vi "MultiChannelFeedback_test_no_before (Host).vi"(5 "RIO Device":T1="RIO0") -> ()   [LabVIEW 2016]
doc: "This VI will will initialize the FPGA VI and then continually read and convert single point values from 4 channels of an analog input module."
uses:
  <vilib>/userdefined/High Color/nirio_resource_hc.ctl
  <vilib>/rvi/Analysis/host/Butterworth/config/Butterworth Filter Order.ctl
  <vilib>/rvi/Analysis/host/Butterworth/config/Butterworth Filter Type.ctl
  <vilib>/FPGAPlugInAG/PXIe-7847R/niLvFpga_Open_PXIe-7847R.vi
  <vilib>/FPGAPlugInAG/PXIe-7847R/niLvFpga_Run_PXIe-7847R.vi
  <vilib>/rvi/Analysis/host/Butterworth/config/BwScaledCoefficients.vi
  <vilib>/Utility/error.llb/Error Cluster From Error Code.vi
  <vilib>/rvi/errors/niLvFpgaAdjustHostInterfaceError.vi
  <vilib>/Utility/file.llb/Read From Spreadsheet File (I64).vi
  <vilib>/FPGAPlugInAG/PXIe-7847R/niLvFpga_Close_PXIe-7847R.vi
  <vilib>/rvi/interface/nirviOpenFPGA/nirviOpenFPGA.xnode
  FPGA Bitfiles/Microspherefeedb_FPGATarget_MultiChannelfFee_-5RO42C0JZ0.lvbitx
  <vilib>/rvi/interface/nirviMethod/nirviMethod.xnode
  <vilib>/rvi/Analysis/host/Butterworth/XNode/ButterworthCoefficients.xnode
  <vilib>/rvi/interface/nirviReadWriteControl/nirviReadWriteControl.xnode
  <vilib>/rvi/interface/nirviCloseFPGA/nirviCloseFPGA.xnode
  NiFpgaLv.dll
  <vilib>/rvi/Analysis/host/Public/NI_FpgaMspHost.lvlib
panel:
  in  "ramp arb drive":bool
  in  "Write data to buffers":bool
  in  "z scale":fxp<+/-,33,17>=1.0
  in  "End value (ch1)":fxp<+/-,32,16>=1.0
  in  "Step (ch1)":fxp<+/-,32,16>=0.100006103515625
  in  "End value (ch0)":fxp<+/-,32,16>=1.0
  in  "Step (ch0)":fxp<+/-,32,16>=1.0
  in  "Delay Time (s)":dbl=0.001
  in  "gain (Z)":fxp<+/-,24,12>=1.0
  in  "steps per cycle":u16=40
  in  "gain (Y)":fxp<+/-,24,12>
  in  "gain (X)":fxp<+/-,24,12>=1.0
  in  "Buffer file path":path=path "C:/Users/UsphereLab/Documents/GitHub/Optlev/scriptssiny_buffer.txt"
  in  "Ramp":bool
  in  "End value power":i16=-800
  in  "Step power":i16=1
  in  "Delay Time (s) power":dbl=0.1 caption="Delay Time (s)"
  in  "LP FF Z":dbl=5000.0
  in  "LP FF Y":dbl=5000.0
  in  "LP FF X":dbl=5000.0
  in  "?":u16(ring)=2 items=["Both", "AOD", "Bead"]
  in  "?":u16(ring)=2 items=["Both", "AOD", "Bead"]
  out "Tot feedback + DC, Z":i16(graph)=80
  out "Individual feedback, Z":cluster{"fb_0":i16, "fb_d0":i16}(graph)={"fb_0"=99, "fb_d0"=99}
  out "AI 2":cluster{"AI1":i16, "AI4":i16}(graph)={"AI1"=301, "AI4"=301}
  out "EOM_amplitude_out":dbl=-6.999694842844065
  in  "EOM_offset (-10 to 10 V)":dbl
  in  "EOM_amplitude (-10 to 10 V)":dbl=-7.0
  in  "EOM_threshold (0 to 1), (2*thr - 1)*ampli":dbl=1.0
  in  "EOM reset":bool
  in  "Pg Y":fxp<+/-,24,12>
  in  "Ig Y":fxp<+/-,24,6>=3.814697265625e-06
  in  "Pg X":fxp<+/-,24,12>
  in  "Ig X":fxp<+/-,24,6>=-3.814697265625e-06
  in  "hp freq Y":dbl=1300.0
  in  "hp freq X":dbl=1300.0
  in  "lp freq X":dbl=1300.0
  in  "DC offset X":i16
  in  "Lower lim X":fxp<+/-,16,16>=-30000.0
  in  "Upper lim X":fxp<+/-,16,16>=30000.0
  in  "Dg X":fxp<+/-,24,12>=-3.5
  in  "X setpoint":i16
  in  "Update":bool
  in  "hp freq Z":dbl=3200.0
  in  "lp freq Y":dbl=1300.0
  in  "lp freq Z":dbl=3200.0
  in  "Count(usec)":u32=10
  in  "?":u16(ring)=2 items=["Both", "AOD", "Bead"]
  in  "?":u16(ring)=2 items=["Both", "AOD", "Bead"]
  in  "?":u16(ring)=2 items=["Both", "AOD", "Bead"]
  in  "?":u16(ring)=2 items=["Both", "AOD", "Bead"]
  in  "Ig Z":fxp<+/-,24,6>=3.814697265625e-06
  in  "DC offset Z":i16=-19
  in  "Lower lim Z":fxp<+/-,16,16>=-700.0
  in  "Upper lim Z":fxp<+/-,16,16>=1500.0
  in  "Dg Z":fxp<+/-,24,12>=3.0
  in  "Pg Z":fxp<+/-,24,12>=0.150146484375
  in  "Z setpoint":i16=300
  in  "Update":bool
  in  "Update":bool
  in  "DC offset Y":i16
  in  "Lower lim Y":fxp<+/-,16,16>=-30000.0
  in  "Upper lim Y":fxp<+/-,16,16>=30000.0
  in  "Dg Y":fxp<+/-,24,12>=6.0
  in  "Y setpoint":i16
  out "Tot feedback + DC, Y":i16(graph)=2990
  out "Individual feedback, Y":cluster{"fb_0":i16, "fb_d0":i16}(graph)={"fb_0"=2990, "fb_d0"=2990}
  out "AI1":cluster{"AI1":i16, "AI4":i16}(graph)={"AI1"=13, "AI4"=13}
  out "Tot feedback + DC, X":i16(graph)=-2975
  out "Individual feedback, X":cluster{"fb_0":i16, "fb_d0":i16}(graph)={"fb_0"=-2975, "fb_d0"=-2975}
  out "AI0":cluster{"AI0":i16, "AI3":i16}(graph)={"AI0"=1, "AI3"=1}
  in  "stop":bool
  # "PID controls, X (AO 0):"
  # "Feedback gains:"
  # "Bandpass filter:"
  # "PID controls, Y (AO 1):"
  # "Feedback gains:"
  # "Bandpass filter:"
  # "PID controls, Z (AO 2):"
  # "Feedback gains:"
  # "Bandpass filter:"
  # "Arb. drive"
  # "Rotation controls (AO3?)"
  # "Ramp control"
types:
  T1 = typedef "nirio_resource_hc.ctl" = tag
  T2 = cluster{"AI X plot":i16, "AI X before chamber plot":i16}
  T3 = cluster{"AI X before chamber plot":i16, "AI X before chamber plot":i16}
  T4 = cluster{"fb X plot":i16, "fb X before chamber plot":i16}
  T5 = cluster{"fb X before chamber plot":i16, "fb X before chamber plot":i16}
  T6 = cluster{"AI Y plot":i16, "AI Y before chamber plot":i16}
  T7 = cluster{"AI Y before chamber plot":i16, "AI Y before chamber plot":i16}
  T8 = cluster{"fb Y plot":i16, "fb Y before chamber plot":i16}
  T9 = cluster{"fb Y before chamber plot":i16, "fb Y before chamber plot":i16}
  T10 = cluster{"AI Z plot":i16, "AI Z before chamber plot":i16}
  T11 = cluster{"AI Z before chamber plot":i16, "AI Z before chamber plot":i16}
  T12 = cluster{"fb Z plot":i16, "fb Z before chamber plot":i16}
  T13 = cluster{"fb Z before chamber plot":i16, "fb Z before chamber plot":i16}
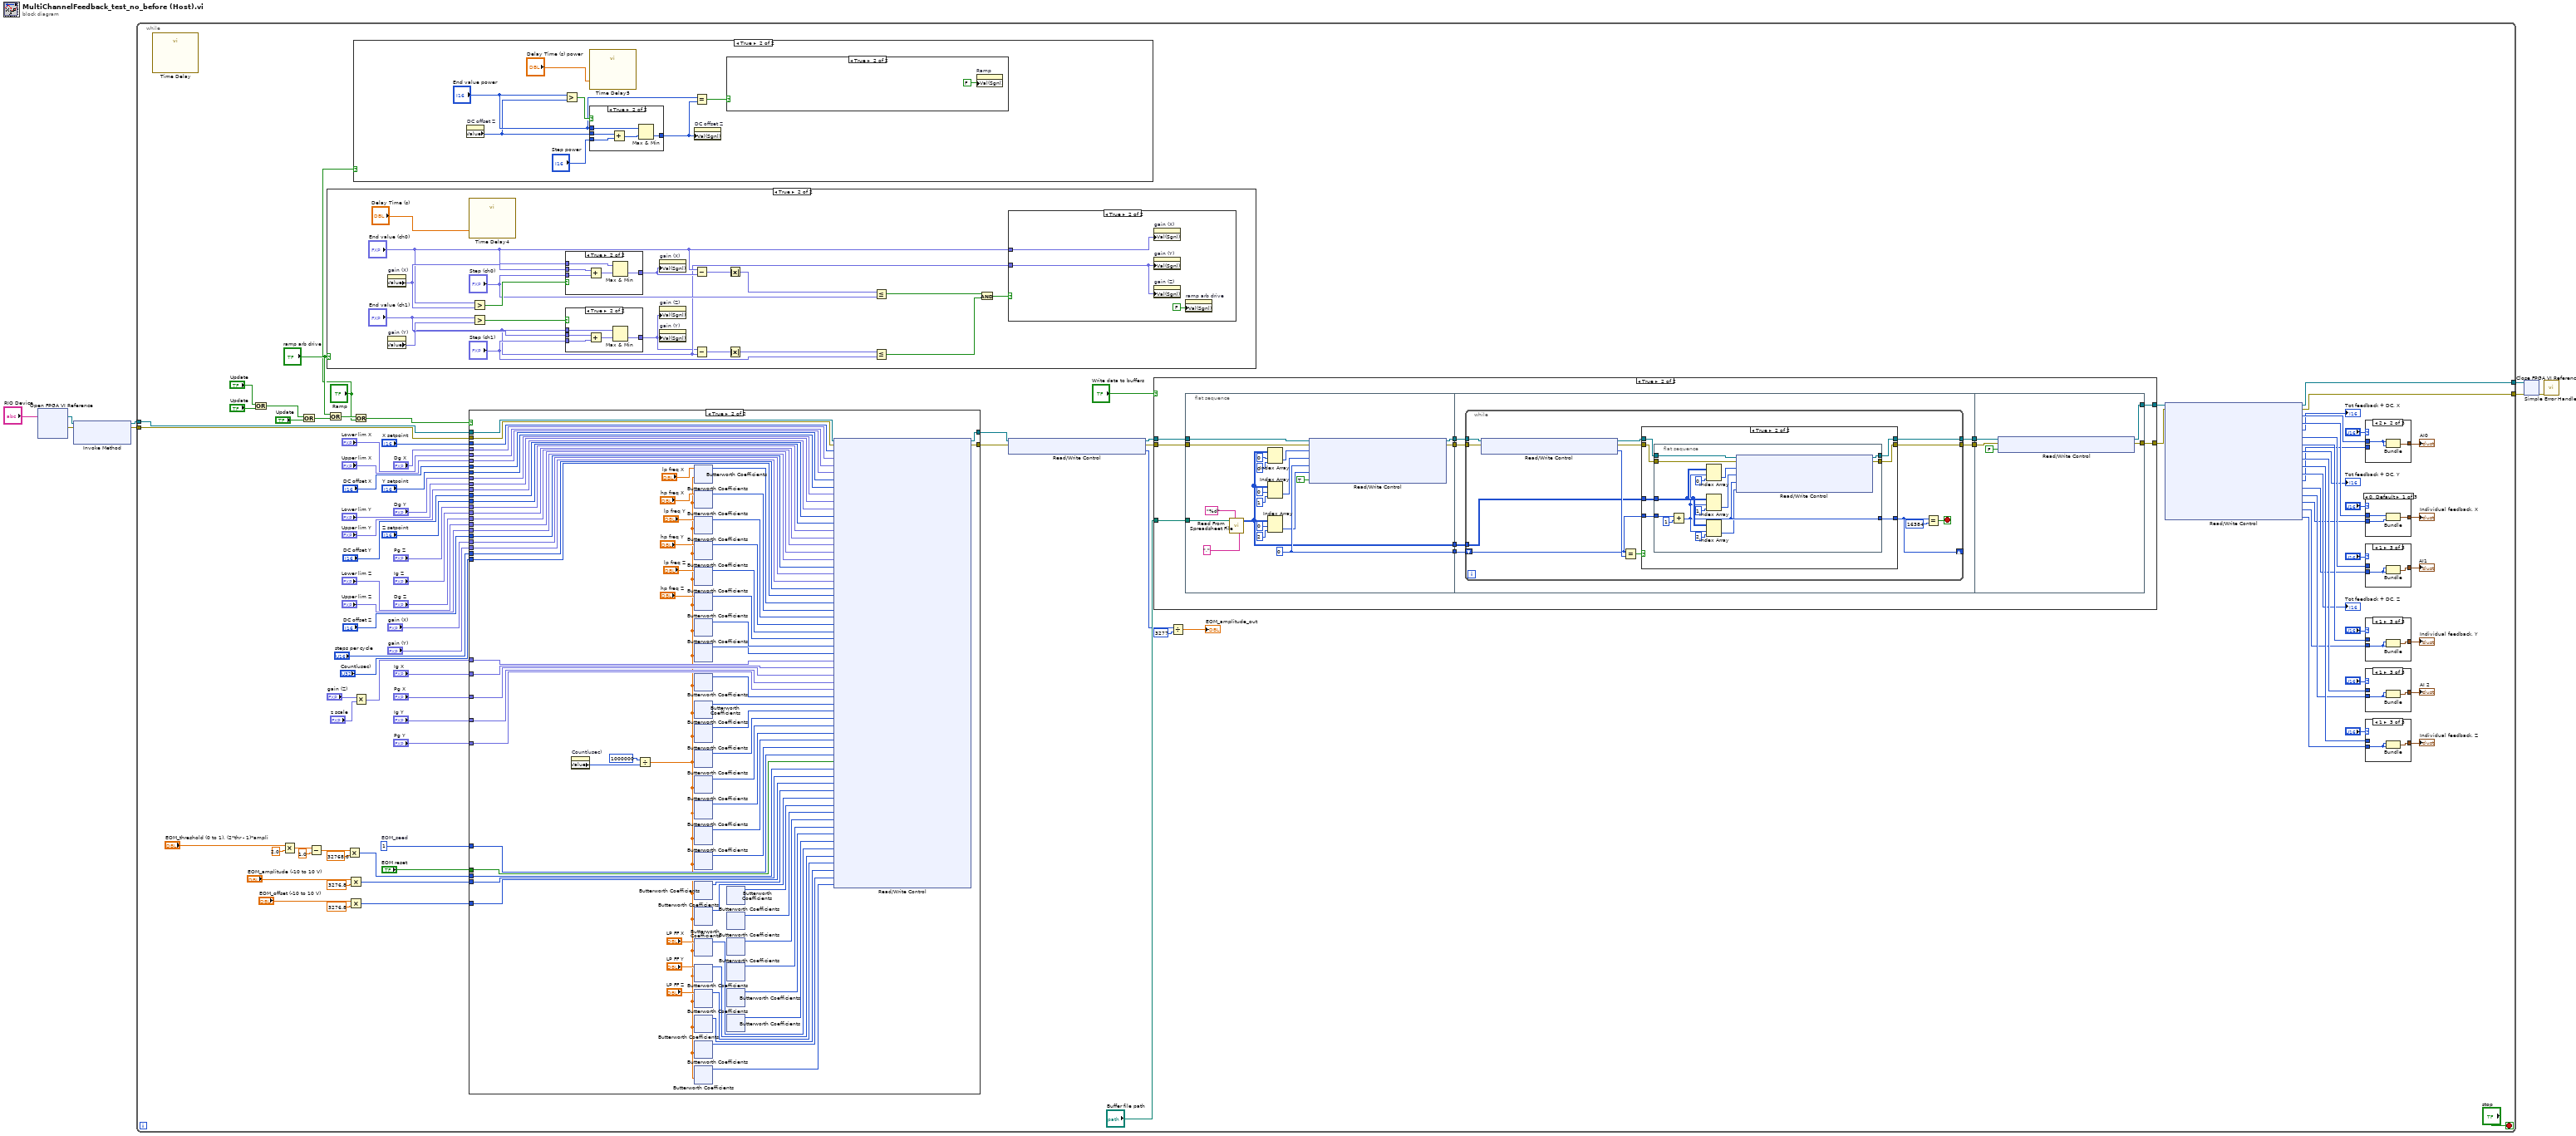
[diagram p0: block diagram]
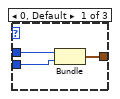
[diagram p2: hidden frame]
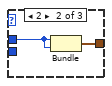
[diagram p3: hidden frame]
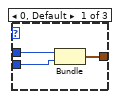
[diagram p4: hidden frame]
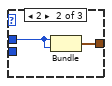
[diagram p5: hidden frame]
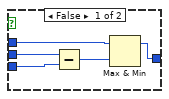
[diagram p8: hidden frame]
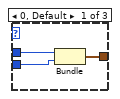
[diagram p9: hidden frame]
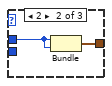
[diagram p10: hidden frame]
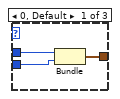
[diagram p11: hidden frame]
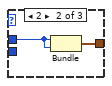
[diagram p12: hidden frame]
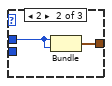
[diagram p13: hidden frame]
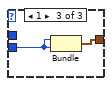
[diagram p14: hidden frame]
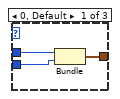
[diagram p15: hidden frame]
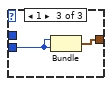
[diagram p16: hidden frame]
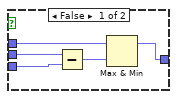
[diagram p18: hidden frame]
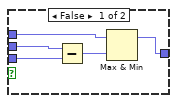
[diagram p20: hidden frame]
diagram:
  n1 = xnode "Open FPGA VI Reference"("resource name"="RIO Device") -> ("FPGA VI Reference Out"=w3:refnum<k20>, "error out"=w2:errorcluster)  [unwired: 1 in]
  n2 = xnode "Invoke Method"("FPGA VI Reference In"=w3, "error in"=w2) -> ("FPGA VI Reference Out"=w5:refnum<k20>, "error out"=w4:errorcluster)  [unwired: 1 in]
  n3 = while {
    tunnel: [w103] -> w8
    tunnel: w5 -> [w95]
    tunnel: w4 -> [w94]
    tunnel: [w102] -> w1
    stop <- "stop" stop-if-true
    w44 = u32 1  # EOM_seed
    n4 = call "Time Delay"() -> ()  [unwired: 11 in, 1 out]
    n5 = Or(x="Update", y="Update") -> (x .or. y?=w73:bool)
    n6 = Multiply(x="EOM_threshold (0 to 1), (2*thr - 1)*ampli", y=2.0) -> (x*y=w40:dbl)
    n7 = Or(x=w73, y="Update") -> (x .or. y?=w53:bool)
    n8 = Subtract(x=w40, y=1.0) -> (x-y=w38:dbl)
    n9 = case shown="True" "ramp arb drive" {
      frame False {
      }
      frame True {
        n10 = property on="gain (X)" class="DigNum (strict)"() -> ("Value"=w180:fxp<+/-,24,12>)  [unwired: 2 in, 2 out]
        n11 = property on="gain (Y)" class="DigNum (strict)"() -> ("Value"=w177:fxp<+/-,24,12>)  [unwired: 2 in, 2 out]
        n12 = call "Time Delay4"("Delay Time (s)"="Delay Time (s)") -> ()  [unwired: 10 in, 1 out]
        n13 = Greater?(x="End value (ch0)", y=w180) -> (0:w181:bool)
        n14 = Greater?(x="End value (ch1)", y=w177) -> (0:w178:bool)
        n15 = case shown="True" w181 {
          tunnel: "End value (ch0)" -> [w196 w201]
          tunnel: w180 -> [w199 w204]
          tunnel: "Step (ch0)" -> [w198 w203]
          tunnel: [w195 w200] -> w176
          frame False {
            n16 = Subtract(x=w199, y=w198) -> (x-y=w197:fxp<+/-,33,17>)
            n17 = Max & Min(x=w196, y=w197) -> (max(x,y)=w195:fxp<+/-,33,17>)  [unwired: 1 out]
          }
          frame True {
            n18 = Add(x=w204, y=w203) -> (x+y=w202:fxp<+/-,33,17>)
            n19 = Max & Min(x=w201, y=w202) -> (min(x,y)=w200:fxp<+/-,33,17>)  [unwired: 1 out]
          }
        }
        n20 = case shown="True" w178 {
          tunnel: "End value (ch1)" -> [w183 w189]
          tunnel: w177 -> [w186 w187]
          tunnel: "Step (ch1)" -> [w185 w191]
          tunnel: [w182 w188] -> w164
          frame False {
            n21 = Subtract(x=w186, y=w185) -> (x-y=w184:fxp<+/-,33,17>)
            n22 = Max & Min(x=w183, y=w184) -> (max(x,y)=w182:fxp<+/-,33,17>)  [unwired: 1 out]
          }
          frame True {
            n23 = Add(x=w187, y=w191) -> (x+y=w190:fxp<+/-,33,17>)
            n24 = Max & Min(x=w189, y=w190) -> (min(x,y)=w188:fxp<+/-,33,17>)  [unwired: 1 out]
          }
        }
        n25 = property on="gain (X)" class="DigNum (strict)"("Val(Sgnl)"=w176) -> ()  [unwired: 2 in, 2 out]
        n26 = property on="gain (Z)" class="DigNum (strict)"("Val(Sgnl)"=w164) -> ()  [unwired: 2 in, 2 out]
        n27 = property on="gain (Y)" class="DigNum (strict)"("Val(Sgnl)"=w164) -> ()  [unwired: 2 in, 2 out]
        n28 = Subtract(x="End value (ch0)", y=w176) -> (x-y=w175:fxp<+/-,34,18>)
        n29 = Subtract(x=w164, y="End value (ch1)") -> (x-y=w172:fxp<+/-,34,18>)
        n30 = Absolute Value(x=w175) -> (abs(x)=w174:fxp<+,33,17>)
        n31 = Absolute Value(x=w172) -> (abs(x)=w171:fxp<+,33,17>)
        n32 = Less Or Equal?(x=w174, y="Step (ch0)") -> (x <= y?=w168:bool)
        n33 = Less Or Equal?(x=w171, y="Step (ch1)") -> (x <= y?=w167:bool)
        n34 = And(x=w168, y=w167) -> (x .and. y?=w169:bool)
        n35 = case shown="True" w169 {
          tunnel: "End value (ch0)" -> [_ w193]
          tunnel: "End value (ch1)" -> [_ w192]
          frame False {
          }
          frame True {
            n36 = property on="gain (X)" class="DigNum (strict)"("Val(Sgnl)"=w193) -> ()  [unwired: 2 in, 2 out]
            n37 = property on="gain (Y)" class="DigNum (strict)"("Val(Sgnl)"=w192) -> ()  [unwired: 2 in, 2 out]
            n38 = property on="gain (Z)" class="DigNum (strict)"("Val(Sgnl)"=w192) -> ()  [unwired: 2 in, 2 out]
            n39 = property on="ramp arb drive" class="Bool (strict)"("Val(Sgnl)"=FALSE) -> ()  [unwired: 2 in, 2 out]
          }
        }
      }
    }
    n40 = Or(x="ramp arb drive", y=w53) -> (x .or. y?=w56:bool)
    n41 = Multiply(x=w38, y=32768.0) -> (x*y=w36:i16)
    n42 = Multiply(x="EOM_amplitude (-10 to 10 V)", y=3276.8) -> (x*y=w33:i16)
    n43 = Multiply(x="EOM_offset (-10 to 10 V)", y=3276.8) -> (x*y=w30:i16)
    n44 = case shown="True" "Ramp" {
      frame False {
      }
      frame True {
        n45 = property on="DC offset Z" class="DigNum (strict)"() -> ("Value"=w119:i16)  [unwired: 2 in, 2 out]
        n46 = Greater?(x="End value power", y=w119) -> (0:w124:bool)
        n47 = call "Time Delay5"("Delay Time (s)"="Delay Time (s) power") -> ()  [unwired: 10 in, 1 out]
        n48 = case shown="True" w124 {
          tunnel: "End value power" -> [w127 w132]
          tunnel: w119 -> [w130 w135]
          tunnel: "Step power" -> [w129 w134]
          tunnel: [w126 w131] -> w118
          frame False {
            n49 = Subtract(x=w130, y=w129) -> (x-y=w128:i16)
            n50 = Max & Min(x=w127, y=w128) -> (max(x,y)=w126:i16)  [unwired: 1 out]
          }
          frame True {
            n51 = Add(x=w135, y=w134) -> (x+y=w133:i16)
            n52 = Max & Min(x=w132, y=w133) -> (min(x,y)=w131:i16)  [unwired: 1 out]
          }
        }
        n53 = Equal?(x="End value power", y=w118) -> (x = y?=w123:bool)
        n54 = property on="DC offset Z" class="DigNum (strict)"("Val(Sgnl)"=w118) -> ()  [unwired: 2 in, 2 out]
        n55 = case shown="True" w123 {
          frame False {
          }
          frame True {
            n56 = property on="Ramp" class="Bool (strict)"("Val(Sgnl)"=FALSE) -> ()  [unwired: 2 in, 2 out]
          }
        }
      }
    }
    n57 = Or(x=w56, y="Ramp") -> (x .or. y?=w57:bool)
    n58 = Multiply(x="gain (Z)", y="z scale") -> (x*y=w50:fxp<+/-,56,28>)
    n59 = case shown="True" w57 {
      tunnel: w94 -> [w286 w355]
      tunnel: [w286 w363] -> w29
      tunnel: [w285 w362] -> w28
      tunnel: "X setpoint" -> [_ w361]
      tunnel: "Dg X" -> [_ w360]
      tunnel: "Upper lim X" -> [_ w358]
      tunnel: "Lower lim X" -> [_ w359]
      tunnel: "DC offset X" -> [_ w357]
      tunnel: w95 -> [w285 w356]
      tunnel: "Y setpoint" -> [_ w354]
      tunnel: "Dg Y" -> [_ w353]
      tunnel: "Lower lim Y" -> [_ w352]
      tunnel: "Upper lim Y" -> [_ w351]
      tunnel: "DC offset Y" -> [_ w350]
      tunnel: "Z setpoint" -> [_ w349]
      tunnel: "Pg Z" -> [_ w348]
      tunnel: "Ig Z" -> [_ w347]
      tunnel: "Dg Z" -> [_ w346]
      tunnel: "Lower lim Z" -> [_ w345]
      tunnel: "Upper lim Z" -> [_ w344]
      tunnel: "DC offset Z" -> [_ w343]
      tunnel: "gain (Y)" -> [_ w332]
      tunnel: "steps per cycle" -> [_ w342]
      tunnel: "Count(usec)" -> [_ w341]
      tunnel: w50 -> [_ w323]
      tunnel: "Ig X" -> [_ w322]
      tunnel: "Pg X" -> [_ w321]
      tunnel: "Ig Y" -> [_ w320]
      tunnel: "Pg Y" -> [_ w319]
      tunnel: w44 -> [_ w310]
      tunnel: "EOM reset" -> [_ w309]
      tunnel: w36 -> [_ w308]
      tunnel: w33 -> [_ w307]
      tunnel: w30 -> [_ w306]
      tunnel: "gain (X)" -> [_ w287]
      frame False {
      }
      frame True {
        n60 = property on="Count(usec)" class="DigNum (strict)"() -> ("Value"=w337:u32)  [unwired: 2 in, 2 out]
        n61 = Divide(x=u32 1000000, y=w337) -> (x/y=w289:dbl)
        n62 = xnode "Butterworth Coefficients"("cutoff frequency (Hz)"="lp freq X", "sample rate (S/s)"=w289) -> ("scaled coefficients"=w331:i32[])  [unwired: 1 in, 1 out]
        n63 = xnode "Butterworth Coefficients"("cutoff frequency (Hz)"="hp freq X", "sample rate (S/s)"=w289) -> ("scaled coefficients"=w330:i32[])  [unwired: 1 in, 1 out]
        n64 = xnode "Butterworth Coefficients"("cutoff frequency (Hz)"="lp freq Y", "sample rate (S/s)"=w289) -> ("scaled coefficients"=w329:i32[])  [unwired: 1 in, 1 out]
        n65 = xnode "Butterworth Coefficients"("cutoff frequency (Hz)"="hp freq Y", "sample rate (S/s)"=w289) -> ("scaled coefficients"=w328:i32[])  [unwired: 1 in, 1 out]
        n66 = xnode "Butterworth Coefficients"("cutoff frequency (Hz)"="lp freq Z", "sample rate (S/s)"=w289) -> ("scaled coefficients"=w327:i32[])  [unwired: 1 in, 1 out]
        n67 = xnode "Butterworth Coefficients"("cutoff frequency (Hz)"="hp freq Z", "sample rate (S/s)"=w289) -> ("scaled coefficients"=w326:i32[])  [unwired: 1 in, 1 out]
        n68 = xnode "Butterworth Coefficients"("sample rate (S/s)"=w289) -> ("scaled coefficients"=w325:i32[])  [unwired: 2 in, 1 out]
        n69 = xnode "Butterworth Coefficients"("sample rate (S/s)"=w289) -> ("scaled coefficients"=w324:i32[])  [unwired: 2 in, 1 out]
        n70 = xnode "Butterworth Coefficients"("sample rate (S/s)"=w289) -> ("scaled coefficients"=w318:i32[])  [unwired: 2 in, 1 out]
        n71 = xnode "Butterworth Coefficients"("sample rate (S/s)"=w289) -> ("scaled coefficients"=w317:i32[])  [unwired: 2 in, 1 out]
        n72 = xnode "Butterworth Coefficients"("sample rate (S/s)"=w289) -> ("scaled coefficients"=w315:i32[])  [unwired: 2 in, 1 out]
        n73 = xnode "Butterworth Coefficients"("sample rate (S/s)"=w289) -> ("scaled coefficients"=w316:i32[])  [unwired: 2 in, 1 out]
        n74 = xnode "Butterworth Coefficients"("sample rate (S/s)"=w289) -> ("scaled coefficients"=w314:i32[])  [unwired: 2 in, 1 out]
        n75 = xnode "Butterworth Coefficients"("sample rate (S/s)"=w289) -> ("scaled coefficients"=w313:i32[])  [unwired: 2 in, 1 out]
        n76 = xnode "Butterworth Coefficients"("sample rate (S/s)"=w289) -> ("scaled coefficients"=w312:i32[])  [unwired: 2 in, 1 out]
        n77 = xnode "Butterworth Coefficients"("sample rate (S/s)"=w289) -> ("scaled coefficients"=w311:i32[])  [unwired: 2 in, 1 out]
        n78 = xnode "Butterworth Coefficients"("sample rate (S/s)"=w289) -> ("scaled coefficients"=w305:i32[])  [unwired: 2 in, 1 out]
        n79 = xnode "Butterworth Coefficients"("sample rate (S/s)"=w289) -> ("scaled coefficients"=w304:i32[])  [unwired: 2 in, 1 out]
        n80 = xnode "Butterworth Coefficients"("cutoff frequency (Hz)"="LP FF X", "sample rate (S/s)"=w289) -> ("scaled coefficients"=w296:i32[])  [unwired: 1 in, 1 out]
        n81 = xnode "Butterworth Coefficients"("cutoff frequency (Hz)"="LP FF Y", "sample rate (S/s)"=w289) -> ("scaled coefficients"=w294:i32[])  [unwired: 1 in, 1 out]
        n82 = xnode "Butterworth Coefficients"("cutoff frequency (Hz)"="LP FF Z", "sample rate (S/s)"=w289) -> ("scaled coefficients"=w292:i32[])  [unwired: 1 in, 1 out]
        n83 = xnode "Butterworth Coefficients"("sample rate (S/s)"=w289) -> ("scaled coefficients"=w291:i32[])  [unwired: 2 in, 1 out]
        n84 = xnode "Butterworth Coefficients"("sample rate (S/s)"=w289) -> ("scaled coefficients"=w290:i32[])  [unwired: 2 in, 1 out]
        n85 = xnode "Butterworth Coefficients"("sample rate (S/s)"=w289) -> ("scaled coefficients"=w288:i32[])  [unwired: 2 in, 1 out]
        n86 = xnode "Butterworth Coefficients"() -> ("scaled coefficients"=w303:i32[])  [unwired: 3 in, 1 out]
        n87 = xnode "Butterworth Coefficients"() -> ("scaled coefficients"=w302:i32[])  [unwired: 3 in, 1 out]
        n88 = xnode "Butterworth Coefficients"() -> ("scaled coefficients"=w301:i32[])  [unwired: 3 in, 1 out]
        n89 = xnode "Butterworth Coefficients"() -> ("scaled coefficients"=w300:i32[])  [unwired: 3 in, 1 out]
        n90 = xnode "Butterworth Coefficients"() -> ("scaled coefficients"=w299:i32[])  [unwired: 3 in, 1 out]
        n91 = xnode "Butterworth Coefficients"() -> ("scaled coefficients"=w298:i32[])  [unwired: 3 in, 1 out]
        n92 = xnode "Read/Write Control"("FPGA VI Reference In"=w356, "error in"=w355, "X Setpoint"=w361, "dg X"=w360, "Lower lim X"=w359, "Upper lim X"=w358, "DC offset X"=w357, "Y Setpoint"=w354, "dg Y"=w353, "Lower lim Y"=w352, "Upper lim Y"=w351, "DC offset Y"=w350, "Z Setpoint"=w349, "pg Z"=w348, "ig Z"=w347, "dg Z"=w346, "Lower lim Z"=w345, "Upper lim Z"=w344, "DC offset Z"=w343, "Arb gain (ch0)"=w287, "Arb gain (ch1)"=w332, "Arb steps per cycle"=w342, "Count(uSec)"=w341, "LP Coeff X"=w331, "HP Coeff X"=w330, "LP Coeff Y"=w329, "HP Coeff Y"=w328, "LP Coeff Z"=w327, "HP Coeff Z"=w326, "LP Coeff band Z before"=w325, "HP coeff band Z before"=w324, "Arb gain (ch2)"=w323, "ig X"=w322, "pg X"=w321, "ig Y"=w320, "pg Y"=w319, "HP Coeff band X"=w318, "LP Coeff band X"=w317, "HP Coeff band Y"=w315, "LP Coeff band Y"=w316, "HP Coeff band Z"=w314, "LP Coeff band Z"=w313, "HP Coeff band Z"=w312, "LP Coeff band Z"=w311, "EOM_seed"=w310, "EOM reset"=w309, "EOM_threshold"=w308, "EOM_amplitude"=w307, "EOM_offset"=w306, "LP Coeff Y before"=w305, "HP Coeff Y before"=w304, "LP Coeff band Y before"=w303, "HP coeff band Y before"=w302, "LP Coeff X before"=w301, "HP Coeff X before"=w300, "LP Coeff band X before"=w299, "HP coeff band X before"=w298, "final filter coeff X"=w296, "final filter coeff Y"=w294, "final filter coeff Z"=w292, "final filter coeff X before"=w291, "final filter coeff Y before"=w290, "final filter coeff Z before"=w288) -> ("FPGA VI Reference Out"=w362:refnum<k20>, "error out"=w363:errorcluster)
      }
    }
    n93 = xnode "Read/Write Control"("FPGA VI Reference In"=w28, "error in"=w29) -> ("FPGA VI Reference Out"=w27:refnum<k20>, "error out"=w26:errorcluster, "EOM_amplitude"=w25:i16)
    n94 = case shown="True" "Write data to buffers" {
      tunnel: "Buffer file path" -> [_ w217]
      tunnel: w27 -> [w206 w216]
      tunnel: w26 -> [w205 w215]
      tunnel: [w206 w208] -> w91
      tunnel: [w205 w207] -> w90
      frame False {
      }
      frame True {
        n95 = flat-sequence {
          tunnel: w217 -> [w236]
          tunnel: w216 -> [w234]
          tunnel: w215 -> [w233]
          tunnel: [w228] -> w214
          tunnel: [w227] -> w213
          tunnel: [w221] -> w212
          tunnel: [w226] -> w211
          tunnel: w214 -> [w242]
          tunnel: w213 -> [w241]
          tunnel: w212 -> [w240]
          tunnel: w211 -> [w239]
          tunnel: [w238] -> w210
          tunnel: [w237] -> w209
          tunnel: w210 -> [w284]
          tunnel: w209 -> [w283]
          tunnel: [w282] -> w208
          tunnel: [w281] -> w207
          frame #0 {
            w226 = 0
            n96 = call-poly <vilib>:"Read From Spreadsheet File.vi"("delimiter (\\t)"="," ("delimiter (\\t)"), "format (%d)"="%d", "file path (dialog if empty)"=w236) -> ("all rows"=w221:i64[][])  [unwired: 4 in, 4 out]
            n97 = Index Array(array=w221, index (row)=0, index (col)=0 ("disabled index (col)")) -> (element=w225:i64)
            n98 = Index Array(array=w221, index (row)=0, index (col)=1 ("disabled index (col)")) -> (element=w224:i64)
            n99 = Index Array(array=w221, index (row)=0, index (col)=2 ("disabled index (col)")) -> (element=w218:i64)
            n100 = xnode "Read/Write Control"("FPGA VI Reference In"=w234, "error in"=w233, "data_buffer_1"=w225, "data_buffer2"=w224, "write_address"=w226, "data_buffer3"=w218, "ready_to_write"=TRUE) -> ("FPGA VI Reference Out"=w227:refnum<k20>, "error out"=w228:errorcluster)
          }
          frame #1 {
            n101 = while {
              shift-right: [w243] -> _
              shift-left: w239 -> [w251]
              tunnel: w241 -> [w255]
              tunnel: w242 -> [w254]
              tunnel: w240 -> [w250]
              tunnel: [w245] -> w238
              tunnel: [w244] -> w237
              stop <- w246 stop-if-true
              n102 = xnode "Read/Write Control"("FPGA VI Reference In"=w255, "error in"=w254) -> ("FPGA VI Reference Out"=w249:refnum<k20>, "error out"=w248:errorcluster, "written_address"=w253:u32)
              n103 = Equal?(x=w251, y=w253) -> (x = y?=w252:bool)
              n104 = case shown="True" w252 {
                tunnel: w251 -> [w258 w265]
                tunnel: w250 -> [_ w264]
                tunnel: w249 -> [w257 w263]
                tunnel: w248 -> [w256 w262]
                tunnel: [w258 w261] -> w243
                tunnel: [w257 w260] -> w245
                tunnel: [w256 w259] -> w244
                frame False {
                }
                frame True {
                  n105 = flat-sequence {
                    tunnel: w265 -> [w278]
                    tunnel: w264 -> [w268]
                    tunnel: w263 -> [w275]
                    tunnel: w262 -> [w274]
                    tunnel: [w267] -> w261
                    tunnel: [w272] -> w260
                    tunnel: [w271] -> w259
                    frame #0 {
                      n106 = Add(x=w278, y=1) -> (x+y=w267:i32)
                      n107 = Index Array(array=w268, index (row)=w267, index (col)=0 ("disabled index (col)")) -> (element=w270:i64)
                      n108 = Index Array(array=w268, index (row)=w267, index (col)=1 ("disabled index (col)")) -> (element=w273:i64)
                      n109 = Index Array(array=w268, index (row)=w267, index (col)=2) -> (element=w266:i64)
                      n110 = xnode "Read/Write Control"("FPGA VI Reference In"=w275, "error in"=w274, "data_buffer_1"=w270, "data_buffer2"=w273, "write_address"=w267, "data_buffer3"=w266) -> ("FPGA VI Reference Out"=w272:refnum<k20>, "error out"=w271:errorcluster)
                    }
                  }
                }
              }
              n111 = Equal?(x=w243, y=u16 16384) -> (x = y?=w246:bool)
            }
          }
          frame #2 {
            n112 = xnode "Read/Write Control"("FPGA VI Reference In"=w284, "error in"=w283, "ready_to_write"=FALSE) -> ("FPGA VI Reference Out"=w282:refnum<k20>, "error out"=w281:errorcluster)
          }
        }
      }
    }
    n113 = Divide(x=w25, y=i16 3277) -> (x/y=→"EOM_amplitude_out":dbl)
    n114 = xnode "Read/Write Control"("FPGA VI Reference In"=w91, "error in"=w90) -> ("FPGA VI Reference Out"=w103:refnum<k20>, "error out"=w102:errorcluster, "AI X plot"=w71:i16, "fb X plot"=w66:i16, "tot_fb X plot"=→"Tot feedback + DC, X":i16, "AI Y plot"=w63:i16, "fb Y plot"=w61:i16, "tot_fb Y plot"=→"Tot feedback + DC, Y":i16, "AI Z plot"=w18:i16, "fb Z plot"=w17:i16, "tot_fb Z plot"=→"Tot feedback + DC, Z":i16, "AI X before chamber plot"=w15:i16, "AI Y before chamber plot"=w14:i16, "AI Z before chamber plot"=w13:i16, "fb X before chamber plot"=w12:i16, "fb Y before chamber plot"=w11:i16, "fb Z before chamber plot"=w10:i16)
    n115 = case shown="2" "?" {
      tunnel: w71 -> [w159 w160 _]
      tunnel: [w158 w161 w163] -> w70
      tunnel: w15 -> [w157 _ w162]
      frame 0, Default {
        n116 = Bundle("AI X plot"=w159, "AI X before chamber plot"=w157) -> (w158:T2)  [unwired: 1 in]
      }
      frame 2 {
        n117 = Bundle("AI X plot"=w160, "AI X plot"=w160) -> (w161:cluster{"AI X plot":i16, "AI X plot":i16})  [unwired: 1 in]
      }
      frame 1 {
        n118 = Bundle("AI X before chamber plot"=w162, "AI X before chamber plot"=w162) -> (w163:T3)  [unwired: 1 in]
      }
    }
    "AI0" <- w70
    n119 = case shown="0, Default" "?" {
      tunnel: w66 -> [w152 w153 _]
      tunnel: [w151 w154 w156] -> w68
      tunnel: w12 -> [w150 _ w155]
      frame 0, Default {
        n120 = Bundle("fb X plot"=w152, "fb X before chamber plot"=w150) -> (w151:T4)  [unwired: 1 in]
      }
      frame 2 {
        n121 = Bundle("fb X plot"=w153, "fb X plot"=w153) -> (w154:cluster{"fb X plot":i16, "fb X plot":i16})  [unwired: 1 in]
      }
      frame 1 {
        n122 = Bundle("fb X before chamber plot"=w155, "fb X before chamber plot"=w155) -> (w156:T5)  [unwired: 1 in]
      }
    }
    "Individual feedback, X" <- w68
    n123 = case shown="1" "?" {
      tunnel: w63 -> [w144 w146 _]
      tunnel: [w145 w147 w149] -> w58
      tunnel: w14 -> [w143 _ w148]
      frame 0, Default {
        n124 = Bundle("AI Y plot"=w144, "AI Y before chamber plot"=w143) -> (w145:T6)  [unwired: 1 in]
      }
      frame 2 {
        n125 = Bundle("AI Y plot"=w146, "AI Y plot"=w146) -> (w147:cluster{"AI Y plot":i16, "AI Y plot":i16})  [unwired: 1 in]
      }
      frame 1 {
        n126 = Bundle("AI Y before chamber plot"=w148, "AI Y before chamber plot"=w148) -> (w149:T7)  [unwired: 1 in]
      }
    }
    "AI1" <- w58
    n127 = case shown="1" "?" {
      tunnel: w61 -> [w137 w139 _]
      tunnel: [w138 w140 w142] -> w60
      tunnel: w11 -> [w136 _ w141]
      frame 0, Default {
        n128 = Bundle("fb Y plot"=w137, "fb Y before chamber plot"=w136) -> (w138:T8)  [unwired: 1 in]
      }
      frame 2 {
        n129 = Bundle("fb Y plot"=w139, "fb Y plot"=w139) -> (w140:cluster{"fb Y plot":i16, "fb Y plot":i16})  [unwired: 1 in]
      }
      frame 1 {
        n130 = Bundle("fb Y before chamber plot"=w141, "fb Y before chamber plot"=w141) -> (w142:T9)  [unwired: 1 in]
      }
    }
    "Individual feedback, Y" <- w60
    n131 = case shown="1" "?" {
      tunnel: w18 -> [w112 w114 _]
      tunnel: [w113 w115 w117] -> w19
      tunnel: w13 -> [w111 _ w116]
      frame 0, Default {
        n132 = Bundle("AI Z plot"=w112, "AI Z before chamber plot"=w111) -> (w113:T10)  [unwired: 1 in]
      }
      frame 2 {
        n133 = Bundle("AI Z plot"=w114, "AI Z plot"=w114) -> (w115:cluster{"AI Z plot":i16, "AI Z plot":i16})  [unwired: 1 in]
      }
      frame 1 {
        n134 = Bundle("AI Z before chamber plot"=w116, "AI Z before chamber plot"=w116) -> (w117:T11)  [unwired: 1 in]
      }
    }
    "AI 2" <- w19
    n135 = case shown="1" "?" {
      tunnel: w17 -> [w105 w107 _]
      tunnel: [w106 w108 w110] -> w20
      tunnel: w10 -> [w104 _ w109]
      frame 0, Default {
        n136 = Bundle("fb Z plot"=w105, "fb Z before chamber plot"=w104) -> (w106:T12)  [unwired: 1 in]
      }
      frame 2 {
        n137 = Bundle("fb Z plot"=w107, "fb Z plot"=w107) -> (w108:cluster{"fb Z plot":i16, "fb Z plot":i16})  [unwired: 1 in]
      }
      frame 1 {
        n138 = Bundle("fb Z before chamber plot"=w109, "fb Z before chamber plot"=w109) -> (w110:T13)  [unwired: 1 in]
      }
    }
    "Individual feedback, Z" <- w20
  }
  n139 = xnode "Close FPGA VI Reference"("FPGA VI Reference In"=w8, "error in"=w1) -> ("error out"=w7:errorcluster)
  n140 = call <vilib>:"Simple Error Handler.vi"("error in (no error)"=w7) -> ()  [unwired: 4 in, 5 out]
